vi "Get Channel Properties.vi"(0 "Item Ref In":T1 format="%.0x", 11 "에러 입력(에러 없음)":errorcluster) -> (1 "Item Ref out":T1 format="%.0x", 2 "Enable Termination Char":bool, 3 "Timeout":u16, 4 "Flow Control":u16, 6 "VISA\nResource\nName":string, 8 "Stop Bits":u16, 10 "Baud rate":u16, 13 "Data bits":u16, 14 "Parity":u16, 15 "에러 출력":errorcluster)   [LabVIEW 2017, in "Serial Communcation Devices Custom Device.lvlib"]
uses:
  Serial Communcation Devices Custom Device.lvlib
  <vilib>/NI Veristand/Custom Device API/Custom Device Item Ref.ctl
  <vilib>/NI Veristand/Custom Device API/Get Item Property (Boolean).vi
  <vilib>/NI Veristand/Custom Device API/Get Item Property (U16).vi
  <vilib>/NI Veristand/Custom Device API/Get Item Property (String).vi
  <vilib>/NI Veristand/Custom Device API/Custom Device API.lvlib
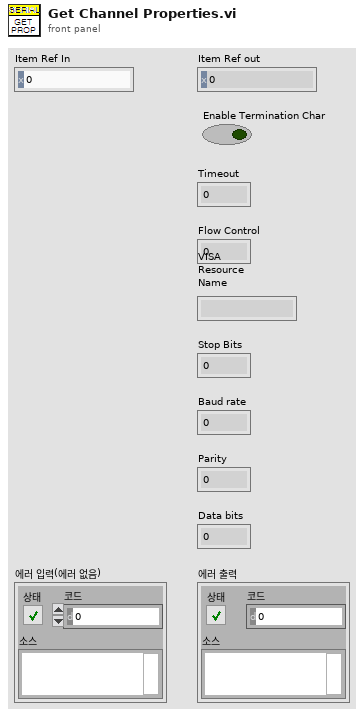
[diagram p1: front panel]
types:
  T1 = typedef "Custom Device API.lvlib/Custom Device Item Ref.ctl" = u64
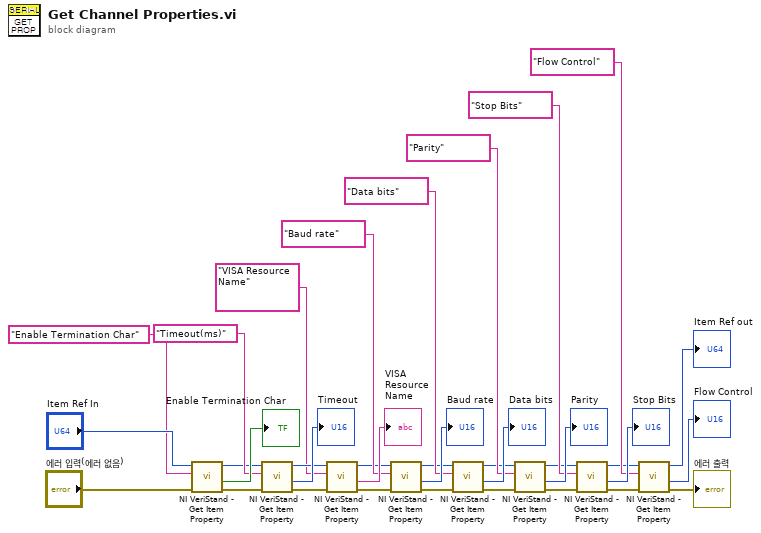
[diagram p0: block diagram]
diagram:
  n1 = call-poly <vilib>:"NI VeriStand - Get Item Property.vi"("error in (no error)"="에러 입력(에러 없음)", "Property Name"="Enable Termination Char", "Item Ref in"="Item Ref In") -> ("error out"=w5:errorcluster, "Value"=→"Enable Termination Char":bool, "Item Ref out"=w4:T1)  [unwired: 5 in, 1 out]
  n2 = call-poly <vilib>:"NI VeriStand - Get Item Property.vi"("error in (no error)"=w5, "Property Name"="Timeout(ms)", "Item Ref in"=w4) -> ("error out"=w6:errorcluster, "Value"=→"Timeout":u16, "Item Ref out"=w19:T1)  [unwired: 5 in, 1 out]
  n3 = call-poly <vilib>:"NI VeriStand - Get Item Property.vi"("error in (no error)"=w6, "Property Name"="VISA Resource Name", "Item Ref in"=w19) -> ("error out"=w7:errorcluster, "Value"=→"VISA\nResource\nName":string, "Item Ref out"=w14:T1)  [unwired: 5 in, 1 out]
  n4 = call-poly <vilib>:"NI VeriStand - Get Item Property.vi"("error in (no error)"=w7, "Property Name"="Baud rate", "Item Ref in"=w14) -> ("error out"=w8:errorcluster, "Value"=→"Baud rate":u16, "Item Ref out"=w15:T1)  [unwired: 5 in, 1 out]
  n5 = call-poly <vilib>:"NI VeriStand - Get Item Property.vi"("error in (no error)"=w8, "Property Name"="Data bits", "Item Ref in"=w15) -> ("error out"=w9:errorcluster, "Value"=→"Data bits":u16, "Item Ref out"=w16:T1)  [unwired: 5 in, 1 out]
  n6 = call-poly <vilib>:"NI VeriStand - Get Item Property.vi"("error in (no error)"=w9, "Property Name"="Parity", "Item Ref in"=w16) -> ("error out"=w10:errorcluster, "Value"=→"Parity":u16, "Item Ref out"=w17:T1)  [unwired: 5 in, 1 out]
  n7 = call-poly <vilib>:"NI VeriStand - Get Item Property.vi"("error in (no error)"=w10, "Property Name"="Stop Bits", "Item Ref in"=w17) -> ("error out"=w11:errorcluster, "Value"=→"Stop Bits":u16, "Item Ref out"=w18:T1)  [unwired: 5 in, 1 out]
  n8 = call-poly <vilib>:"NI VeriStand - Get Item Property.vi"("error in (no error)"=w11, "Property Name"="Flow Control", "Item Ref in"=w18) -> ("error out"=→"에러 출력":errorcluster, "Value"=→"Flow Control":u16, "Item Ref out"=→"Item Ref out":T1)  [unwired: 5 in, 1 out]
